vi "ProjToJson.vi"(8 "error in":errorcluster, 9 "Application ref":refnum<vi>, 10 "Output Directory":path, 11 "LVProj Path":path) -> (0 "error out":errorcluster, 2 "Items To Serialize":T1[](array[typedef]), 3 "JSON":string)   [LabVIEW 2017]
uses:
  ApplicationItems.ctl
  SourceJsonPaths.ctl
  Helpers/DirectoryMetadata/DirectoryMetadata.lvclass
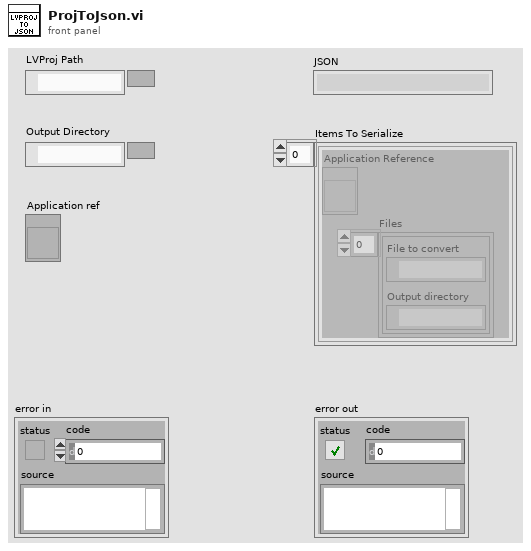
[diagram p1: front panel]
types:
  T1 = typedef "ApplicationItems.ctl" = cluster{"Application Reference":refnum<vi>, "Files":T2[]}
  T2 = typedef "SourceJsonPaths.ctl" = cluster{"File to convert":path, "Output directory":path}
  T3 = cluster{"Context.GetFromProj":refnum<vi>, "Paths":cluster{"Path":path, "JSON Path":path}[]}
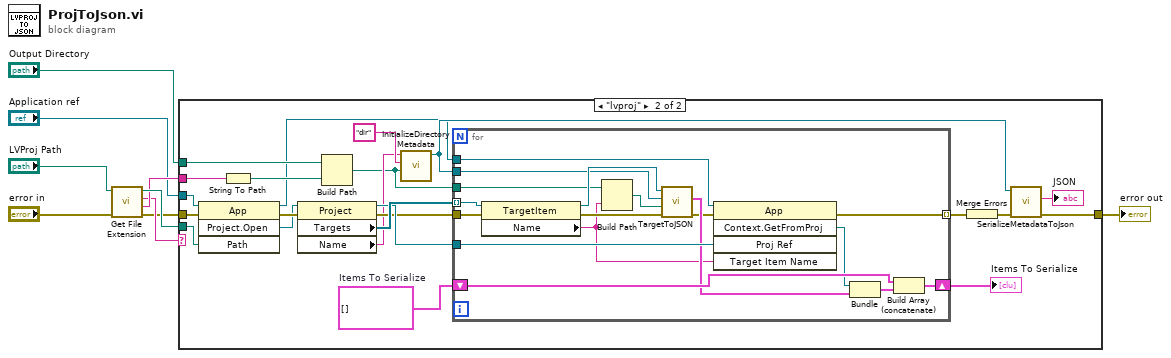
[diagram p0: block diagram]
diagram:
  n1 = call <vilib>:"Get File Extension.vi"("error in (no error)"="error in", "file"="LVProj Path") -> ("error out"=w3:errorcluster, "filename without extension"=w5:string, "lowercase file extension"=w4:string, "dup file"=w7:path)  [unwired: 5 in, 1 out]
  n2 = case shown="\"lvproj\"" w4 {
    tunnel: w7 -> [_ w13]
    tunnel: "Output Directory" -> [_ w15]
    tunnel: w5 -> [_ w18]
    tunnel: w3 -> [w10 w32]
    tunnel: [w10 w19] -> w2
    tunnel: "Application ref" -> [_ w12]
    frame "False", Default {
    }
    frame "lvproj" {
      w31 = T1[] []  # Items To Serialize
      n3 = invoke class="App" method="Project.Open"(reference=w12, error in=w32, "Path"=w13) -> (reference out=w11:refnum<vi>, error out=w30:errorcluster, "Project:Open"=w14:refnum<vi>)  [unwired: 1 in, 1 out]
      n4 = String To Path(string=w18) -> (path=w17:path)
      n5 = property class="Project"(reference=w14, error in=w30) -> (reference out=w28:refnum<vi>, error out=w25:errorcluster, "Targets"=w29:refnum<vi>[], "Name"=w23:string)
      n6 = Build Path(base path=w15, name or relative path=w17) -> (appended path=w16:path)
      n7 = call "InitializeDirectoryMetadata.vi"("Path"=w16, "Type"="dir", "ID"=w23) -> ("DirectoryMetadata instance"=w21:refnum<data-value>)  [unwired: 7 in, 1 out]
      n8 = for {
        tunnel: w16 -> [w35]
        shift-right: [w45] -> w27
        shift-left: w31 -> [w46]
        tunnel: w29 -> [w48] mode=indexing
        tunnel: w28 -> [w49]
        tunnel: [w40] -> w26 mode=indexing
        tunnel: w25 -> [w38]
        tunnel: w21 -> [w37]
        tunnel: w11 -> [w33]
        n9 = property class="TargetItem"(reference=w48, error in=w38) -> (reference out=w47:refnum<vi>, error out=w39:errorcluster, "Name"=w36:string)
        n10 = Build Path(base path=w35, name or relative path=w36) -> (appended path=w34:path)
        n11 = call "TargetToJSON.vi"("error in"=w39, "JSON Path"=w34, "head in"=w37, "Target Obj"=w47) -> ("error out"=w41:errorcluster, "Paths"=w43:cluster{"Path":path, "JSON Path":path}[])  [unwired: 6 in]
        n12 = invoke class="App" method="Context.GetFromProj"(reference=w33, error in=w41, "Proj Ref"=w49, "Target Item Name"=w36) -> (error out=w40:errorcluster, "Context.GetFromProj"=w44:refnum<vi>)  [unwired: 1 in, 3 out]
        n13 = Bundle("Context.GetFromProj"=w44, "Paths"=w43) -> (w42:T3)  [unwired: 1 in]
        n14 = Build Array (concatenate)(w46, w42) -> (w45:T1[])
      }
      "Items To Serialize" <- w27
      n15 = Merge Errors(w26) -> (w20:errorcluster)
      n16 = call "SerializeMetadataToJson.vi"("error in (no error)"=w20, "head in"=w21) -> ("error out"=w19:errorcluster, "Serialized String"=→"JSON":string)  [unwired: 7 in, 1 out]
    }
  }
  "error out" <- w2
